vi "gate_control.vi"() -> ()   [LabVIEW 2016]
uses:
  <instrlib>/Keithley 24XX/Public/Data/Read (Single Point).vi
  <instrlib>/Keithley 24XX/Keithley 24XX.lvlib
panel:
  in  "voltage limit":dbl=70.0
  in  "step":dbl=0.1
  in  "target voltae":dbl
  out "current":sgl(graph)
  out "voltage":sgl(graph)
  out "Voltage":sgl
  out "Current":sgl
  in  "VISA resource name":refnum<visa-resource-name>="GPIB0::27::INSTR"
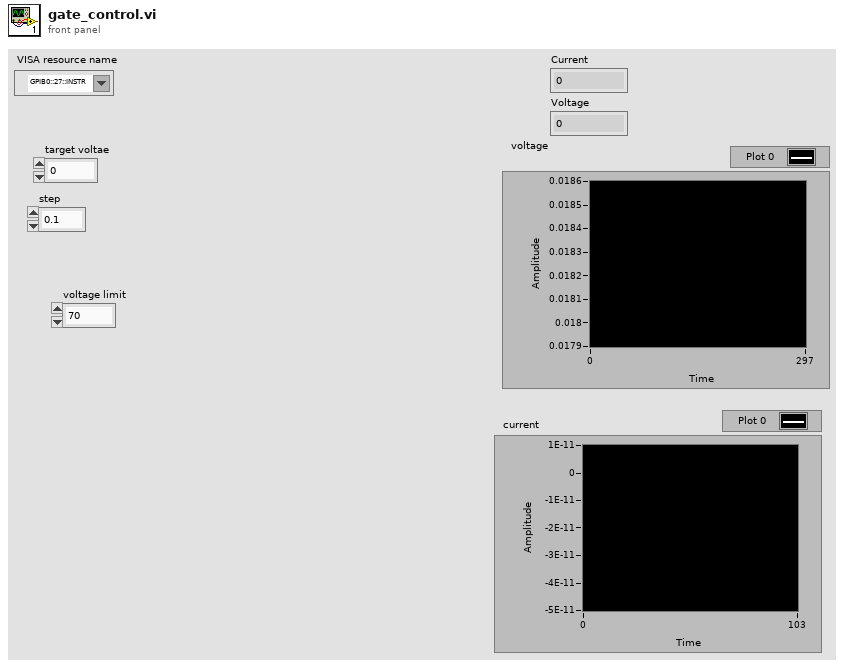
[diagram p1: front panel]
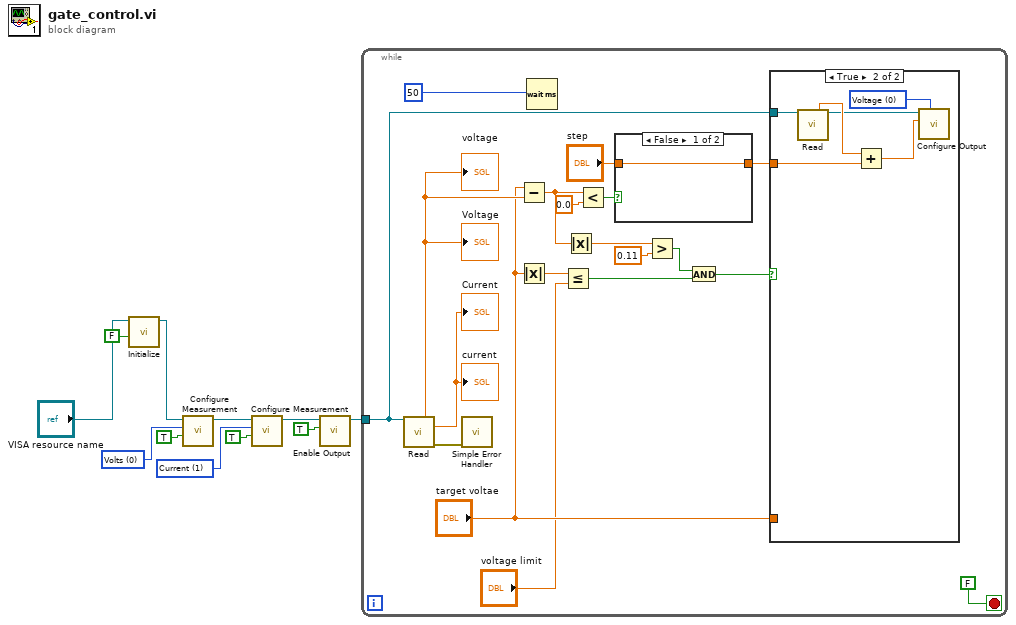
[diagram p0: block diagram]
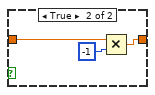
[diagram p2: hidden frame]
diagram:
  w8 = u16 1 items=["Volts", "Current", "Resistance"] ("Function (0: Volts)")
  w9 = u16 0 items=["Volts", "Current", "Resistance"] ("Function (0: Volts)")
  n1 = call <instrlib>:"Initialize.vi"("Reset (True)"=FALSE, "VISA resource name"="VISA resource name") -> ("VISA resource name out"=w1:refnum<visa-resource-name>)  [unwired: 8 in, 1 out]
  n2 = call <instrlib>:"Configure Measurement.vi"("Enable Auto Range (T:Enable)"=TRUE, "Function (0: Volts)"=w9, "VISA resource name"=w1) -> ("VISA resource name out"=w10:refnum<visa-resource-name>)  [unwired: 7 in, 1 out]
  n3 = call <instrlib>:"Configure Measurement.vi"("Enable Auto Range (T:Enable)"=TRUE, "Function (0: Volts)"=w8, "VISA resource name"=w10) -> ("VISA resource name out"=w7:refnum<visa-resource-name>)  [unwired: 7 in, 1 out]
  n4 = call <instrlib>:"Enable Output.vi"("Enable Output (T: Enable)"=TRUE, "VISA resource name"=w7) -> ("VISA resource name out"=w6:refnum<visa-resource-name>)  [unwired: 8 in, 1 out]
  n5 = while {
    tunnel: w6 -> [w27]
    stop <- FALSE stop-if-true
    n6 = call-poly <instrlib>:"Read.vi"("VISA resource name"=w27) -> ("Voltage"=w26:sgl, "Current"=→"Current" →"current":sgl, "error out"=w29:errorcluster)  [unwired: 8 in, 4 out]
    "Voltage" <- w26
    "voltage" <- w26
    n7 = call <vilib>:"Simple Error Handler.vi"("error in (no error)"=w29) -> ()  [unwired: 4 in, 5 out]
    n8 = Subtract(x="target voltae", y=w26) -> (x-y=w17:dbl)
    n9 = Absolute Value(x="target voltae") -> (abs(x)=w22:dbl)
    n10 = Wait (ms)(milliseconds to wait=u32 50 ("millisecond multiple")) -> ()  [unwired: 1 out]
    n11 = Less Or Equal?(x=w22, y="voltage limit") -> (x <= y?=w19:bool)
    n12 = Absolute Value(x=w17) -> (abs(x)=w25:dbl)
    n13 = Less?(x=w17, y=0.0) -> (x < y?=w15:bool)
    n14 = case shown="False" w15 {
      tunnel: "step" -> [w31 w34]
      tunnel: [w31 w32] -> w13
      frame False {
      }
      frame True {
        n15 = Multiply(x=w34, y=-1) -> (x*y=w32:dbl)
      }
    }
    n16 = Greater?(x=w25, y=0.11) -> (0:w20:bool)
    n17 = And(x=w20, y=w19) -> (x .and. y?=w18:bool)
    n18 = case shown="True" w18 {
      tunnel: "target voltae" -> [_ _]
      tunnel: w27 -> [_ w40]
      tunnel: w13 -> [_ w38]
      frame False {
      }
      frame True {
        w37 = u16 0 items=["Voltage", "Current"] ("Source Mode  (0: Voltage)")
        n19 = call-poly <instrlib>:"Read.vi"("VISA resource name"=w40) -> ("Voltage"=w39:sgl, "VISA resource name out"=w36:refnum<visa-resource-name>)  [unwired: 8 in, 5 out]
        n20 = Add(x=w39, y=w38) -> (x+y=w35:dbl)
        n21 = call <instrlib>:"Configure Output.vi"("Source Mode  (0: Voltage)"=w37, "Output Level (0)"=w35, "VISA resource name"=w36) -> ()  [unwired: 7 in, 2 out]
      }
    }
  }
